vi "GlobalSetLaserEmissionOnOffInterlook.vi"() -> ()   [LabVIEW 2011]
panel:
  in  "LaserPower":i32 min=0 max=100 step=1
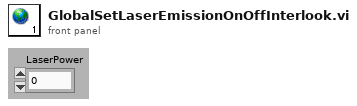
[diagram p1: front panel]
diagram:
